vi "Interval Timer v2 (SubVI).vi"(10 "Interval Time":i32, 11 "Sampling Time":i32) -> ()   [LabVIEW 2019]
doc: "Nested interval timer. Input requires 2 time values in minutes:\n1. Sampling time (X) - length of time to save data (duty cycle TRUE)\n2. Interval (Y) - overall time interval (Y-X = duty cycle FALSE)\n\nY must be greater than X\n\nExample: If X = 7 and Y = 15, The \"Save Raw Data\" boolean global variable will be TRUE for 7 minutes and false for 8 minutes, totalling a 15 miniute interval. After the Y interval expires, the processes is repeated.\n\n2020 NREL"
uses:
  Globals and Definitions/RT Globals RD v1.0.vi
  Globals and Definitions/Initialization Globals.vi
panel:
  out "Snooze Expired":bool
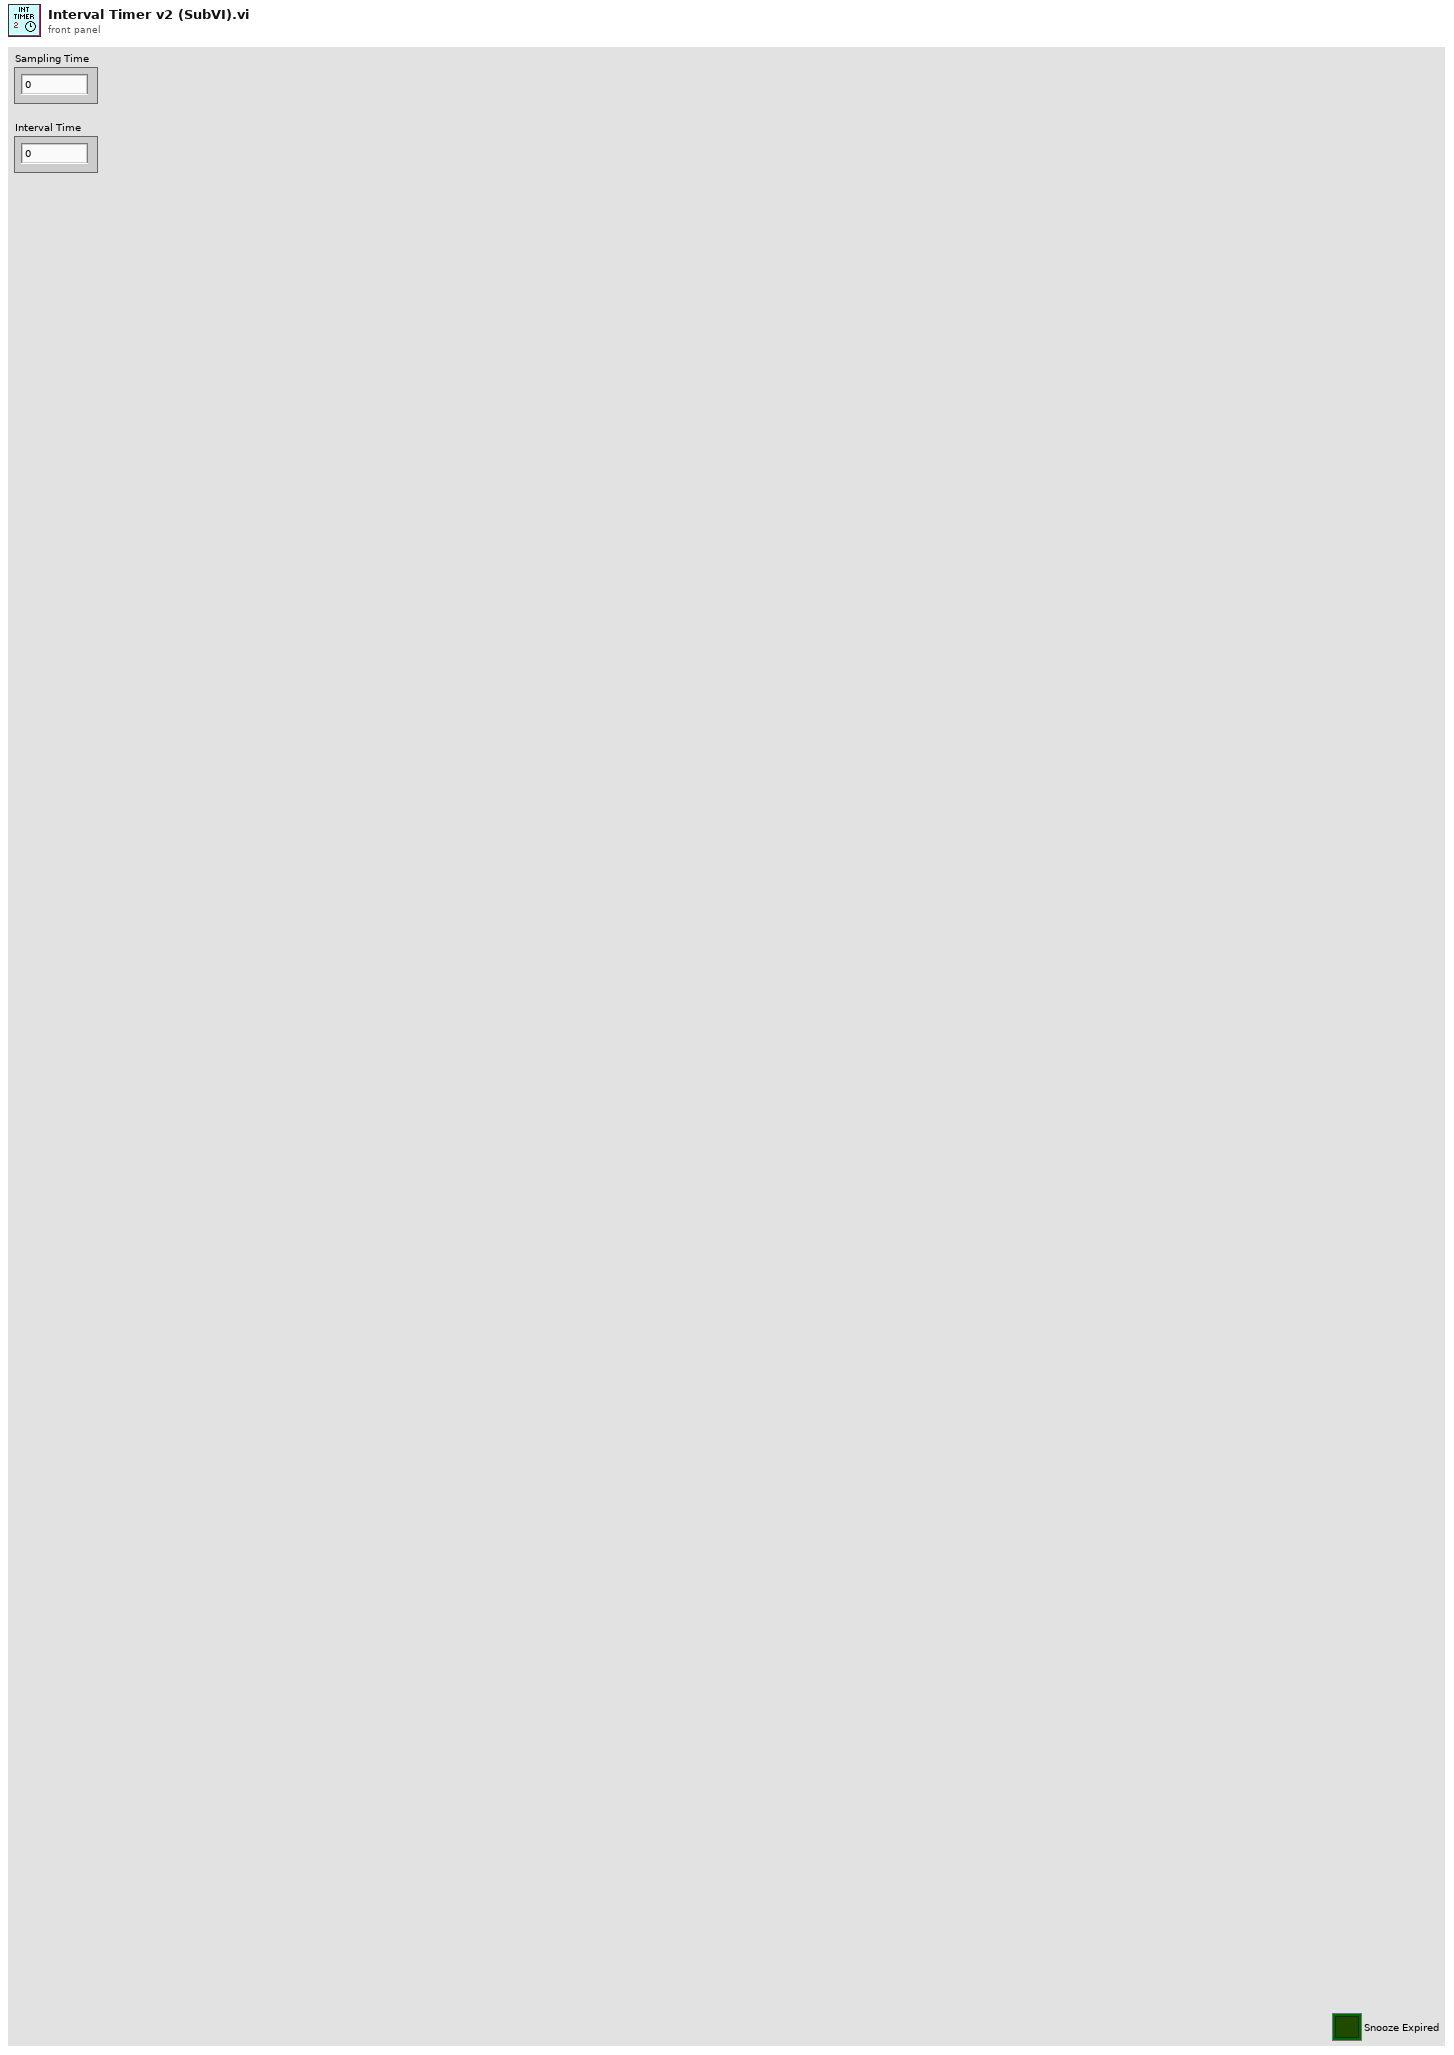
[diagram p1: front panel]
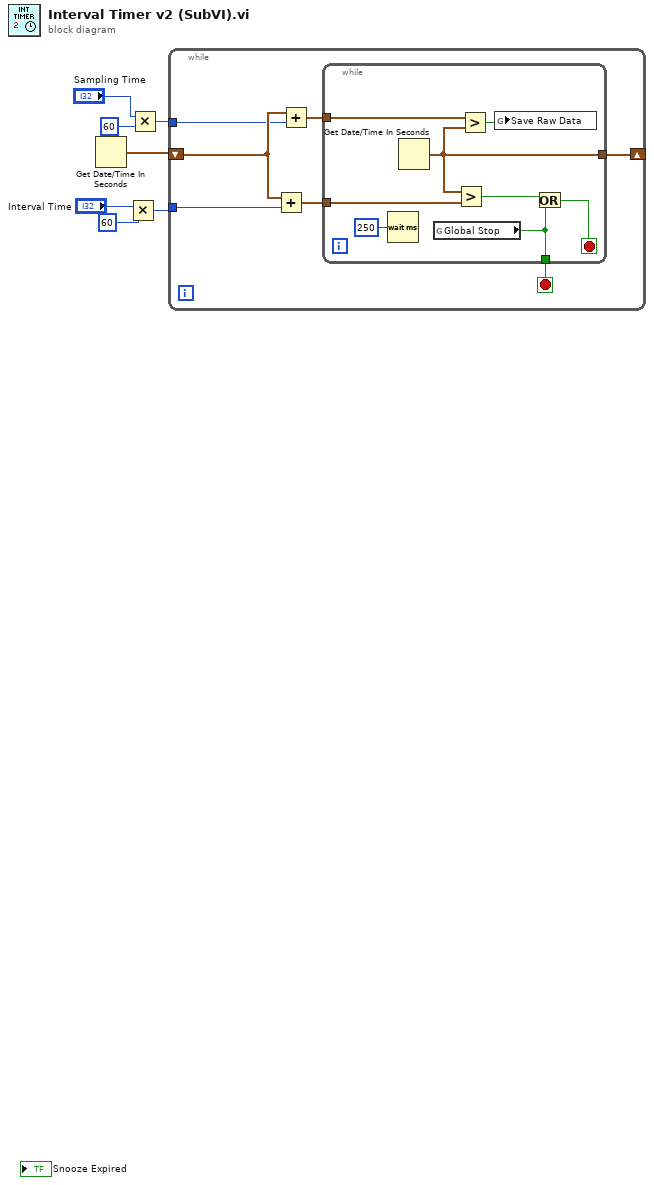
[diagram p0: block diagram]
diagram:
  n1 = Get Date/Time In Seconds() -> (seconds since 1Jan1904=w7:timestamp)
  n2 = Multiply(x="Interval Time", y=60) -> (x*y=w4:i32)
  n3 = Multiply(x="Sampling Time", y=60) -> (x*y=w3:i32)
  n4 = while {
    tunnel: w4 -> [w14]
    tunnel: w3 -> [w12]
    shift-right: [w11] -> _
    shift-left: w7 -> [w13]
    stop <- w10 stop-if-true
    n5 = Add(x=w13, y=w14) -> (x+y=w8:timestamp)
    n6 = Add(x=w13, y=w12) -> (x+y=w9:timestamp)
    n7 = while {
      tunnel: [w21] -> w11
      tunnel: [w15] -> w10
      tunnel: w9 -> [w18]
      tunnel: w8 -> [w17]
      stop <- w19 stop-if-true
      n8 = Wait (ms)(milliseconds to wait=u32 250) -> ()  [unwired: 1 out]
      n9 = Get Date/Time In Seconds() -> (seconds since 1Jan1904=w21:timestamp)
      n10 = global read "RT Globals RD v1.0.vi" "Global Stop"() -> (w15:bool)
      n11 = Greater?(x=w21, y=w17) -> (0:w20:bool)
      n12 = Greater?(x=w18, y=w21) -> (0:w16:bool)
      n13 = global write "Initialization Globals.vi" "Save Raw Data"(w16) -> ()
      n14 = Or(x=w20, y=w15) -> (x .or. y?=w19:bool)
    }
  }
